vi "Byte Buffer.Read.Typed Double Array.vi"(0 "Byte Buffer in":refnum<class "Byte Buffer.lvclass">, 1 "data type":T1, 5 "buffer in":dbl[](array[numeric]), 7 "count":i64, 9 "buffer offset":u64, 11 "error in (no error)":errorcluster) -> (4 "Byte Buffer out":refnum<class "Byte Buffer.lvclass">, 6 "buffer out":dbl[](array[numeric]), 10 "new buffer offset":u64, 15 "error out":errorcluster)   [LabVIEW 2016, in "VeriStand Data.lvlib" / "Byte Buffer.lvclass"]
doc: "Reads <B>count</B> number of elements of the specified <B>data type</B> from the <B>Byte Buffer</B> at the specified <B>buffer offset</B> and converts the values to double floats before writing them to the provided double float <B>buffer</B>."
uses:
  Byte Buffer.lvclass
  Typedefs/Typedefs.Data Types.ctl
  Byte Buffer.lvclass/Byte Buffer.ctl
  Byte Buffer.Read (1D Boolean).vi
  Type Conversion/Type Conversion.To Double.Subset (1D Boolean).vi
  Byte Buffer.Read (1D SGL).vi
  Type Conversion/Type Conversion.To Double.Subset (1D SGL).vi
  Byte Buffer.Read (1D DBL).vi
  Byte Buffer.Read (1D I8).vi
  Type Conversion/Type Conversion.To Double.Subset (1D I8).vi
  Byte Buffer.Read (1D I16).vi
  Type Conversion/Type Conversion.To Double.Subset (1D I16).vi
  Byte Buffer.Read (1D I32).vi
  Type Conversion/Type Conversion.To Double.Subset (1D I32).vi
  Byte Buffer.Read (1D I64).vi
  Type Conversion/Type Conversion.To Double.Subset (1D I64).vi
  Byte Buffer.Read (1D U8).vi
  Type Conversion/Type Conversion.To Double.Subset (1D U8).vi
  Byte Buffer.Read (1D U16).vi
  Type Conversion/Type Conversion.To Double.Subset (1D U16).vi
  Byte Buffer.Read (1D U32).vi
  Type Conversion/Type Conversion.To Double.Subset (1D U32).vi
  Byte Buffer.Read (1D U64).vi
  Type Conversion/Type Conversion.To Double.Subset (1D U64).vi
  Byte Buffer.Read.Typed String.vi
  Type Conversion/Type Conversion.To Double.vi
  Type Conversion/Type Conversion.To Double (1D Boolean).vi
  Type Conversion/Type Conversion.To Double (1D SGL).vi
  Type Conversion/Type Conversion.To Double (1D I8).vi
  Type Conversion/Type Conversion.To Double (1D I16).vi
  Type Conversion/Type Conversion.To Double (1D I32).vi
  Type Conversion/Type Conversion.To Double (1D I64).vi
  Type Conversion/Type Conversion.To Double (1D U8).vi
  Type Conversion/Type Conversion.To Double (1D U16).vi
  Type Conversion/Type Conversion.To Double (1D U32).vi
  Type Conversion/Type Conversion.To Double (1D U64).vi
  Byte Buffer.Subset.Get.vi
  Utilities/Utilities.Sizeof.Array.vi
  Utilities/Utilities.Buffer.String.vi
  Memory Management/Memory Management.MoveByteBlock.Write (String).vi
  Utilities/Utilities.Sizeof.Scalar.vi
  Memory Management/Memory Management.Handle Return.vi
  VeriStand Data.lvlib
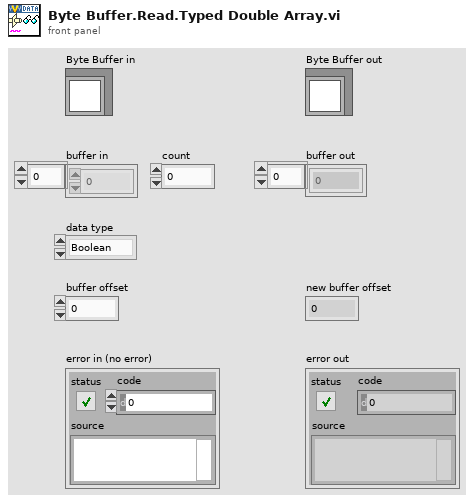
[diagram p1: front panel]
types:
  T1 = typedef "VeriStand Data.lvlib/Typedefs.Data Types.ctl" = enum16{"Boolean", "Single", "Double", "I8", "I16", "I32", "I64", "U8", "U16", "U32", "U64"}
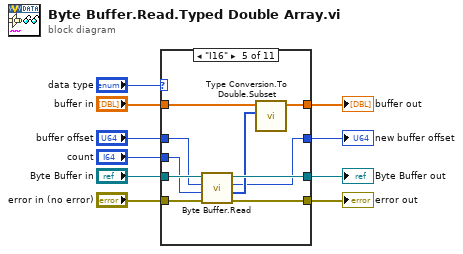
[diagram p0: block diagram]
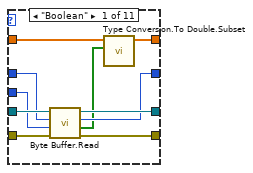
[diagram p2: hidden frame]
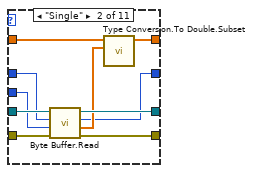
[diagram p3: hidden frame]
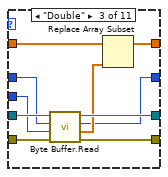
[diagram p4: hidden frame]
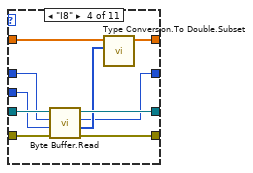
[diagram p5: hidden frame]
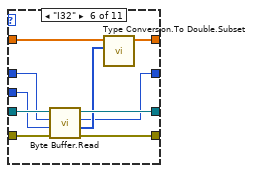
[diagram p6: hidden frame]
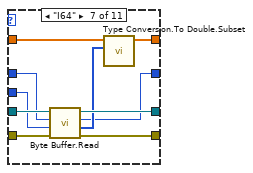
[diagram p7: hidden frame]
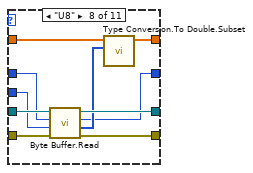
[diagram p8: hidden frame]
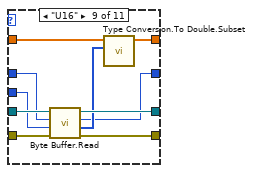
[diagram p9: hidden frame]
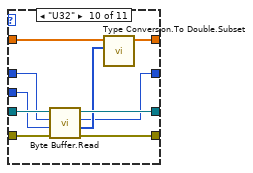
[diagram p10: hidden frame]
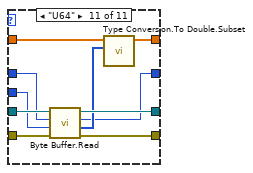
[diagram p11: hidden frame]
diagram:
  n1 = case shown="\"I16\"" "data type" {
    tunnel: "buffer offset" -> [w13 w22 w32 w49 w59 w69 w79 w89 w99 w109 w119]
    tunnel: "Byte Buffer in" -> [w20 w30 w40 w50 w60 w70 w80 w90 w100 w110 w120]
    tunnel: [w14 w24 w36 w43 w53 w63 w73 w83 w93 w103 w113] -> w9
    tunnel: "error in (no error)" -> [w19 w29 w39 w48 w58 w68 w78 w88 w98 w108 w118]
    tunnel: [w17 w27 w37 w46 w56 w66 w76 w86 w96 w106 w116] -> w7
    tunnel: "count" -> [w18 w28 w38 w47 w57 w67 w77 w87 w97 w107 w117]
    tunnel: [w16 w26 w34 w45 w55 w65 w75 w85 w95 w105 w115] -> w6
    tunnel: "buffer in" -> [w15 w25 w35 w44 w54 w64 w74 w84 w94 w104 w114]
    tunnel: [w12 w21 w31 w41 w51 w61 w71 w81 w91 w101 w111] -> w1
    frame "Boolean" {
      n2 = call-poly "Byte Buffer.Read.vi"("error in (no error)"=w19, "count"=w18, "buffer offset"=w13, "Byte Buffer in"=w20) -> ("error out"=w17:errorcluster, "value"=w11:bool[], "new buffer offset"=w12:u64, "Byte Buffer out"=w14:refnum<class "Byte Buffer.lvclass">)  [unwired: 4 in]
      n3 = call-poly "Type Conversion.To Double.Subset.vi"("new values"=w11, "values in"=w15) -> ("values out"=w16:dbl[])  [unwired: 9 in]
    }
    frame "Single" {
      n4 = call-poly "Byte Buffer.Read.vi"("error in (no error)"=w29, "count"=w28, "buffer offset"=w22, "Byte Buffer in"=w30) -> ("error out"=w27:errorcluster, "value"=w23:sgl[], "new buffer offset"=w21:u64, "Byte Buffer out"=w24:refnum<class "Byte Buffer.lvclass">)  [unwired: 4 in]
      n5 = call-poly "Type Conversion.To Double.Subset.vi"("new values"=w23, "values in"=w25) -> ("values out"=w26:dbl[])  [unwired: 9 in]
    }
    frame "Double" {
      n6 = call-poly "Byte Buffer.Read.vi"("error in (no error)"=w39, "count"=w38, "buffer offset"=w32, "Byte Buffer in"=w40) -> ("error out"=w37:errorcluster, "value"=w33:dbl[], "new buffer offset"=w31:u64, "Byte Buffer out"=w36:refnum<class "Byte Buffer.lvclass">)  [unwired: 4 in]
      n7 = Replace Array Subset(array=w35, new element=w33) -> (w34:dbl[])  [unwired: 1 in]
    }
    frame "I8" {
      n8 = call-poly "Byte Buffer.Read.vi"("error in (no error)"=w48, "count"=w47, "buffer offset"=w49, "Byte Buffer in"=w50) -> ("error out"=w46:errorcluster, "value"=w42:i8[], "new buffer offset"=w41:u64, "Byte Buffer out"=w43:refnum<class "Byte Buffer.lvclass">)  [unwired: 4 in]
      n9 = call-poly "Type Conversion.To Double.Subset.vi"("new values"=w42, "values in"=w44) -> ("values out"=w45:dbl[])  [unwired: 9 in]
    }
    frame "I16" {
      n10 = call-poly "Byte Buffer.Read.vi"("error in (no error)"=w58, "count"=w57, "buffer offset"=w59, "Byte Buffer in"=w60) -> ("error out"=w56:errorcluster, "value"=w52:i16[], "new buffer offset"=w51:u64, "Byte Buffer out"=w53:refnum<class "Byte Buffer.lvclass">)  [unwired: 4 in]
      n11 = call-poly "Type Conversion.To Double.Subset.vi"("new values"=w52, "values in"=w54) -> ("values out"=w55:dbl[])  [unwired: 9 in]
    }
    frame "I32" {
      n12 = call-poly "Byte Buffer.Read.vi"("error in (no error)"=w68, "count"=w67, "buffer offset"=w69, "Byte Buffer in"=w70) -> ("error out"=w66:errorcluster, "value"=w62:i32[], "new buffer offset"=w61:u64, "Byte Buffer out"=w63:refnum<class "Byte Buffer.lvclass">)  [unwired: 4 in]
      n13 = call-poly "Type Conversion.To Double.Subset.vi"("new values"=w62, "values in"=w64) -> ("values out"=w65:dbl[])  [unwired: 9 in]
    }
    frame "I64" {
      n14 = call-poly "Byte Buffer.Read.vi"("error in (no error)"=w78, "count"=w77, "buffer offset"=w79, "Byte Buffer in"=w80) -> ("error out"=w76:errorcluster, "value"=w72:i64[], "new buffer offset"=w71:u64, "Byte Buffer out"=w73:refnum<class "Byte Buffer.lvclass">)  [unwired: 4 in]
      n15 = call-poly "Type Conversion.To Double.Subset.vi"("new values"=w72, "values in"=w74) -> ("values out"=w75:dbl[])  [unwired: 9 in]
    }
    frame "U8" {
      n16 = call-poly "Byte Buffer.Read.vi"("error in (no error)"=w88, "count"=w87, "buffer offset"=w89, "Byte Buffer in"=w90) -> ("error out"=w86:errorcluster, "value"=w82:u8[], "new buffer offset"=w81:u64, "Byte Buffer out"=w83:refnum<class "Byte Buffer.lvclass">)  [unwired: 4 in]
      n17 = call-poly "Type Conversion.To Double.Subset.vi"("new values"=w82, "values in"=w84) -> ("values out"=w85:dbl[])  [unwired: 9 in]
    }
    frame "U16" {
      n18 = call-poly "Byte Buffer.Read.vi"("error in (no error)"=w98, "count"=w97, "buffer offset"=w99, "Byte Buffer in"=w100) -> ("error out"=w96:errorcluster, "value"=w92:u16[], "new buffer offset"=w91:u64, "Byte Buffer out"=w93:refnum<class "Byte Buffer.lvclass">)  [unwired: 4 in]
      n19 = call-poly "Type Conversion.To Double.Subset.vi"("new values"=w92, "values in"=w94) -> ("values out"=w95:dbl[])  [unwired: 9 in]
    }
    frame "U32" {
      n20 = call-poly "Byte Buffer.Read.vi"("error in (no error)"=w108, "count"=w107, "buffer offset"=w109, "Byte Buffer in"=w110) -> ("error out"=w106:errorcluster, "value"=w102:u32[], "new buffer offset"=w101:u64, "Byte Buffer out"=w103:refnum<class "Byte Buffer.lvclass">)  [unwired: 4 in]
      n21 = call-poly "Type Conversion.To Double.Subset.vi"("new values"=w102, "values in"=w104) -> ("values out"=w105:dbl[])  [unwired: 9 in]
    }
    frame "U64" {
      n22 = call-poly "Byte Buffer.Read.vi"("error in (no error)"=w118, "count"=w117, "buffer offset"=w119, "Byte Buffer in"=w120) -> ("error out"=w116:errorcluster, "value"=w112:u64[], "new buffer offset"=w111:u64, "Byte Buffer out"=w113:refnum<class "Byte Buffer.lvclass">)  [unwired: 4 in]
      n23 = call-poly "Type Conversion.To Double.Subset.vi"("new values"=w112, "values in"=w114) -> ("values out"=w115:dbl[])  [unwired: 9 in]
    }
  }
  "error out" <- w7
  "Byte Buffer out" <- w9
  "new buffer offset" <- w1
  "buffer out" <- w6
